vi "EmergencyStopAll.vi"() -> ()   [LabVIEW 2016]
uses:
  GenericDriveCommand.ctl
  DriveConfigGlobal.vi
  Anemometry/Anemometry Sub Vis/Globals/Trav_pos_global.vi
panel:
  out "Live Position":dbl[](array[numeric]) format="%.2f"
  in  "stop":bool
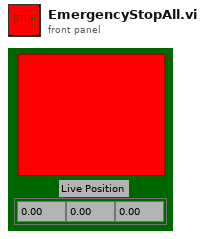
[diagram p1: front panel]
types:
  T1 = typedef "GenericDriveCommand.ctl" = string
  T2 = typedef "AxisConfigCluster.ctl" = cluster{"Channel Properties":T3, "Static Drive Configuration":T4}
  T3 = typedef "DriveProperties.ctl" = cluster{"Channel Name":string, "Vel. Default":sgl, "Acc. Default":sgl, "Vel. Max":sgl, "Vel. Min":sgl, "Acc. Max":sgl, "Acc. Min":sgl, "Pulses/unit":sgl, "Address":u8, "Pulse Offset":i32, "Pos Tolerance":sgl, "Pulses/rev":sgl, "Backlash/Eng units":sgl, "Current Pos":sgl, "Ch Status":enum16{"Active", "Offline", "Simulate"}, "Port Name":string, "Axis Transform mode":string, "Metadata Ch Name":string, "Type":string}
  T4 = typedef "DriveStaticConfig.ctl" = cluster{"Correction Gain % (CG)":u16, "Dead Band (DB)":i32, "Dead Band Window (DW)":i32, "Encoder Resolution (ER)":i32, "Step Mode  (FSB)":u16, "Position Maintenance (FSC)":u16, "Stop on Stall (FSD)":u16, "Activate OP1 on stall (FSE)":u16, "Stop on Trigger 3 (FSF)":u16, "OP2 in Deadband (FSG)":u16, "Stall Detect (FSH)":u16, "Limit Disable (LD)":u16, "Motor Resolution (MR)":enum16{"200", "400", "1000", "2000", "4000", "5000", "10000", "12800", "18000", "20000", "21600", "25000", "25400", "25600", "36000", "50000", "278528", "425984", "507904", "614400", "655360", "819200", "1024000"}, "Limit Switch Sense (OSA)":u16, "Home Position (OSB)":u16, "Home Switch Sense (OSC)":u16, "Encoder Z for Home (OSD)":u16, "Reference edge of Home (OSH)":u16, "RS232 Echo Control (SSA)":u16, "Buffer at Limit (SSG)":u16, "Buffer at Stop (SSH)":u16, "Indexer Mode  (FSA)":u16, "Type":string, "ConfigString":string, "De Power Motor":enum16{"TRUE", "FALSE"}}
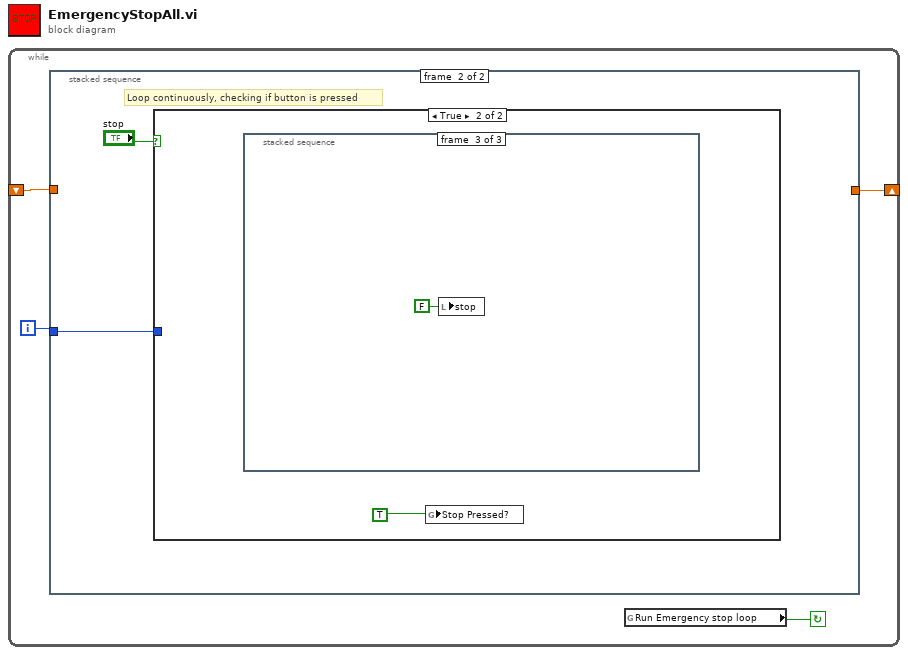
[diagram p0: block diagram]
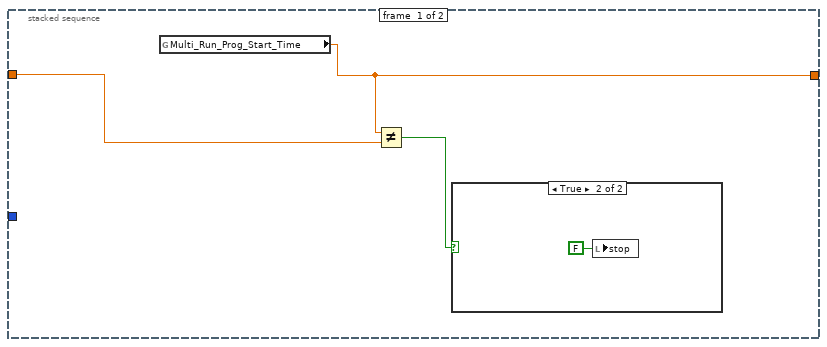
[diagram p2: hidden frame]
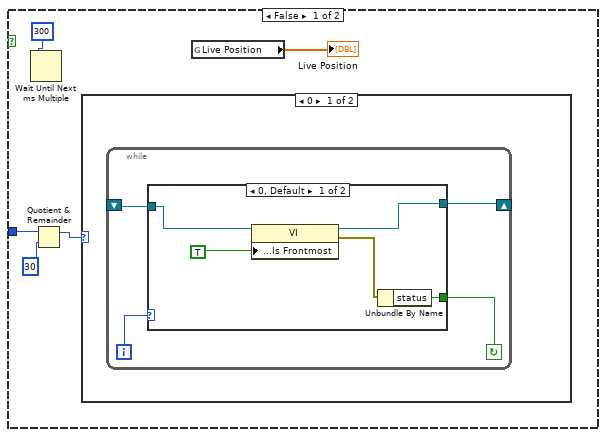
[diagram p4: hidden frame]
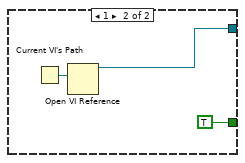
[diagram p5: hidden frame]
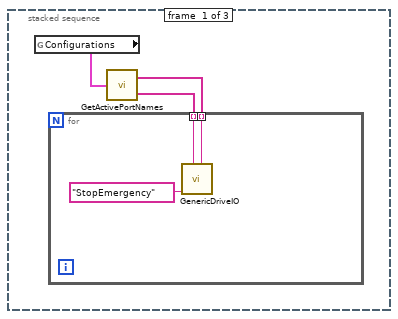
[diagram p7: hidden frame]
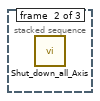
[diagram p8: hidden frame]
diagram:
  n1 = while {
    shift-right: [w2] -> _
    shift-left: _ -> [w1]
    i -> [w3]
    stop <- w4 continue-if-true
    n2 = stacked-sequence {
      tunnel: w3 -> [_ w9]
      tunnel: [w7 _] -> w2
      tunnel: w1 -> [w6 _]
      frame #0 {
        n3 = global read "Trav_pos_global.vi" "Multi_Run_Prog_Start_Time"() -> (w7:dbl)
        n4 = Not Equal?(x=w7, y=w6) -> (x != y?=w5:bool)
        n5 = case shown="True" w5 {
          frame False {
          }
          frame True {
            n6 = local write "stop"(FALSE ("stop")) -> ()
          }
        }
      }
      frame #1 {
        # "Loop continuously, checking if button is pressed"
        n7 = case shown="True" "stop" {
          tunnel: w9 -> [w14 _]
          frame False {
            n8 = Wait Until Next ms Multiple(millisecond multiple=300) -> ()  [unwired: 1 out]
            n9 = Quotient & Remainder(x=w14, y=30) -> (x-y*floor(x/y)=w12:i32)  [unwired: 1 out]
            n10 = case shown="0" w12 {
              frame 0 {
                n11 = while {
                  shift-left: _ -> [w19]
                  shift-right: [w16] -> _
                  i -> [w18]
                  stop <- w17 continue-if-true
                  n12 = case shown="0, Default" w18 {
                    tunnel: w19 -> [w23 _]
                    tunnel: [w21 TRUE ("status")] -> w17
                    tunnel: [w20 w26] -> w16
                    frame 0, Default {
                      n13 = property class="VI"(reference=w23, "Front Panel Window:Is Frontmost"=TRUE) -> (reference out=w20:refnum<vi>, error out=w22:errorcluster)  [unwired: 1 in]
                      n14 = Unbundle By Name(w22) -> ("status"=w21:bool)
                    }
                    frame 1 {
                      n15 = Current VI's Path() -> (path=w27:path)
                      n16 = Open VI Reference(vi path=w27) -> (vi reference=w26:refnum<vi>)  [unwired: 5 in, 1 out]
                    }
                  }
                }
              }
              frame 1, Default {
              }
            }
            n17 = global read "Trav_pos_global.vi" "Live Position"() -> (→"Live Position":sgl[])
          }
          frame True {
            n18 = stacked-sequence {
              frame #0 {
                n19 = global read "DriveConfigGlobal.vi" "Configurations"() -> (w31:T2[])
                n20 = call "GetActivePortNames.vi"("Matched Configurations In"=w31) -> ("Port Name Array"=w30:string[], "Drive Type Array"=w29:string[])
                n21 = for {
                  tunnel: w30 -> [w34] mode=indexing
                  tunnel: w29 -> [w32] mode=indexing
                  n22 = call "GenericDriveIO.vi"("GenericDriveCommand"=T1 "StopEmergency", "Type"=w32, "Port Name"=w34) -> ()  [unwired: 7 in, 2 out]
                }
              }
              frame #1 {
                n23 = call "Shut_down_all_Axis.vi"() -> ()  [unwired: 1 in]
              }
              frame #2 {
                n24 = local write "stop"(FALSE ("stop")) -> ()
              }
            }
            n25 = global write "DriveConfigGlobal.vi" "Stop Pressed?"(TRUE) -> ()
          }
        }
      }
    }
    n26 = global read "DriveConfigGlobal.vi" "Run Emergency stop loop"() -> (w4:bool)
  }
